vi "interupt.vi"(5 "Motor":i32, 6 "error in":errorcluster, 7 "Motor Poisition":cluster{"Go Home":bool, "Position":dbl[]}, 8 "Data Change":bool, 9 "VISA resource In":refnum<visa-resource-name>) -> (0 "error out":errorcluster, 2 "VISA resource name out":refnum<visa-resource-name>)   [LabVIEW 2016]
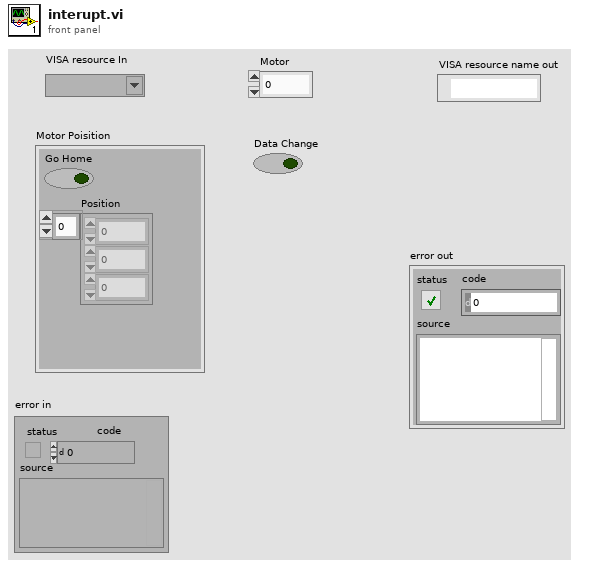
[diagram p1: front panel]
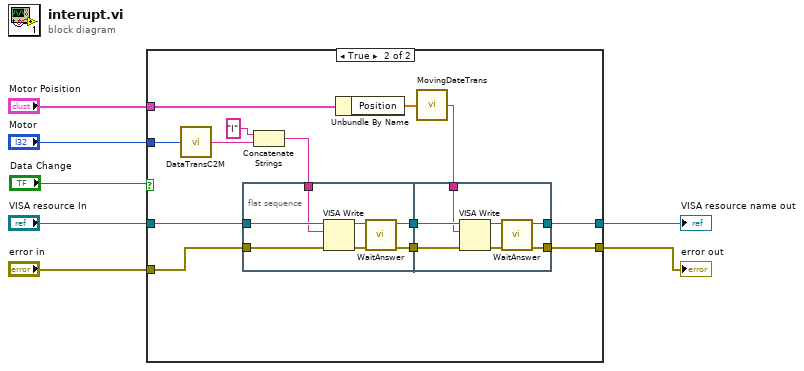
[diagram p0: block diagram]
diagram:
  n1 = case shown="True" "Data Change" {
    tunnel: [w9 w20] -> w7
    tunnel: [w8 w19] -> w6
    tunnel: "VISA resource In" -> [w9 w18]
    tunnel: "error in" -> [w8 w17]
    tunnel: "Motor" -> [_ w16]
    tunnel: "Motor Poisition" -> [_ w10]
    frame False {
    }
    frame True {
      n2 = call "DataTransC2M.vi"("input"=w16) -> ("output"=w13:string)
      n3 = flat-sequence {
        tunnel: w18 -> [w27]
        tunnel: w17 -> [w29]
        tunnel: [w28] -> w22
        tunnel: [w23] -> w21
        tunnel: w12 -> [w25]
        tunnel: w22 -> [w35]
        tunnel: w21 -> [w34]
        tunnel: [w33] -> w20
        tunnel: [w30] -> w19
        tunnel: w11 -> [w32]
        frame #0 {
          n4 = VISA Write(VISA resource name=w27, write buffer=w25, error in (no error)=w29) -> (VISA resource name out=w26:refnum<visa-resource-name>, error out=w24:errorcluster)  [unwired: 1 out]
          n5 = call "WaitAnswer.vi"("error in (no error)"=w24, "VISA resource name in"=w26) -> ("error out"=w23:errorcluster, "VISA resource name out"=w28:refnum<visa-resource-name>)  [unwired: 4 in]
        }
        frame #1 {
          n6 = VISA Write(VISA resource name=w35, write buffer=w32, error in (no error)=w34) -> (VISA resource name out=w36:refnum<visa-resource-name>, error out=w31:errorcluster)  [unwired: 1 out]
          n7 = call "WaitAnswer.vi"("error in (no error)"=w31, "VISA resource name in"=w36) -> ("error out"=w30:errorcluster, "VISA resource name out"=w33:refnum<visa-resource-name>)  [unwired: 4 in]
        }
      }
      n8 = Concatenate Strings("I" ("string"), w13) -> (w12:string)
      n9 = Unbundle By Name(w10) -> ("Position"=w15:dbl[])
      n10 = call "MovingDateTrans.vi"("INPUT"=w15) -> ("MOVEING COMMAND"=w11:string)  [unwired: 2 in]
    }
  }
  "error out" <- w6
  "VISA resource name out" <- w7
